vi "svx_DAQ_TimingCaptionValues.vi"(11 "Timing Mode":T1) -> (0 "Timing Indicator 1 Caption":string, 1 "Timing Control 3 Caption":string, 2 "Timing Control 2 Caption":string, 3 "Timing Control 1 Caption":string, 5 "Timing Control 3 Visible?":bool)   [LabVIEW 2017, in "SVX NI-DAQmx AI Configuration XControl.xctl"]
uses:
  <vilib>/addons/Sound and Vibration/svt_DAQmx/Configuration XControl/SVX NI-DAQmx AI Configuration XControl.xctl
  <vilib>/addons/Sound and Vibration/svt_DAQmx/Configuration XControl/Controls/svx_DAQ_TimingType.ctl
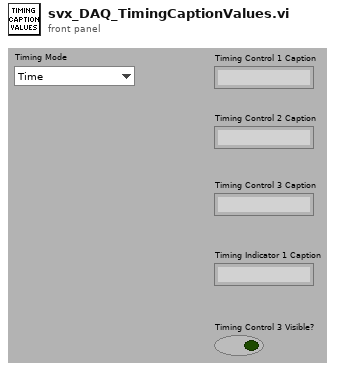
[diagram p1: front panel]
types:
  T1 = typedef "SVX NI-DAQmx AI Configuration XControl.xctl/svx_DAQ_TimingType.ctl" = enum16{"Time", "Frequency", "Order"}
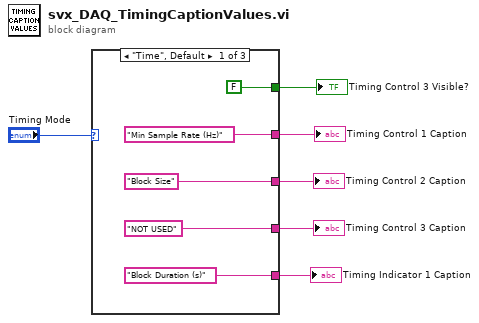
[diagram p0: block diagram]
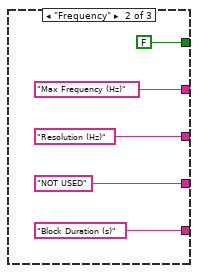
[diagram p2: hidden frame]
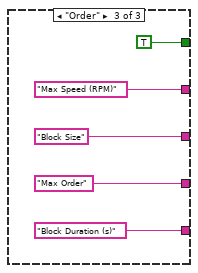
[diagram p3: hidden frame]
diagram:
  n1 = case shown="\"Time\", Default" "Timing Mode" {
    tunnel: ["Min Sample Rate (Hz)" "Max Frequency (Hz)" "Max Speed (RPM)"] -> w2
    tunnel: ["Block Size" "Resolution (Hz)" "Block Size"] -> w3
    tunnel: ["NOT USED" "NOT USED" "Max Order"] -> w4
    tunnel: ["Block Duration (s)" "Block Duration (s)" "Block Duration (s)"] -> w5
    tunnel: [FALSE ("Visible") FALSE ("Visible") TRUE ("Visible")] -> w6
    frame "Time", Default {
    }
    frame "Frequency" {
    }
    frame "Order" {
    }
  }
  "Timing Control 3 Visible?" <- w6
  "Timing Indicator 1 Caption" <- w5
  "Timing Control 3 Caption" <- w4
  "Timing Control 2 Caption" <- w3
  "Timing Control 1 Caption" <- w2
